vi "CopyVI.vi"(8 "error in (no error)":errorcluster, 9 "application reference (local)":refnum<vi>, 10 "Empty File":path=path "D:/Git/CSPP_MessageMaker/_CSPP_MessageMaker/TestVIs/TestTarget.vi", 11 "File to Copy":path) -> (0 "error out":errorcluster)   [LabVIEW 2014]
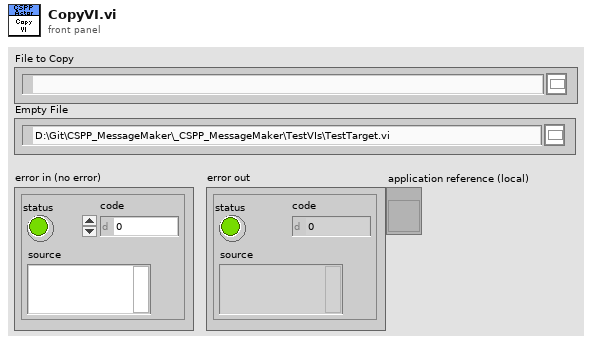
[diagram p1: front panel]
types:
  T1 = enum16{"Invalid Wire Rule", "Required", "Recommended", "Optional", "Dynamic Dispatch"}
  T2 = enum16{"Invalid Wire Rule", "Required", "Recommended", "Optional", "Dynamic Dispatch"}[]
  T3 = typedef "LVPositionTypeDef.ctl" = cluster{"Left":i32, "Top":i32}
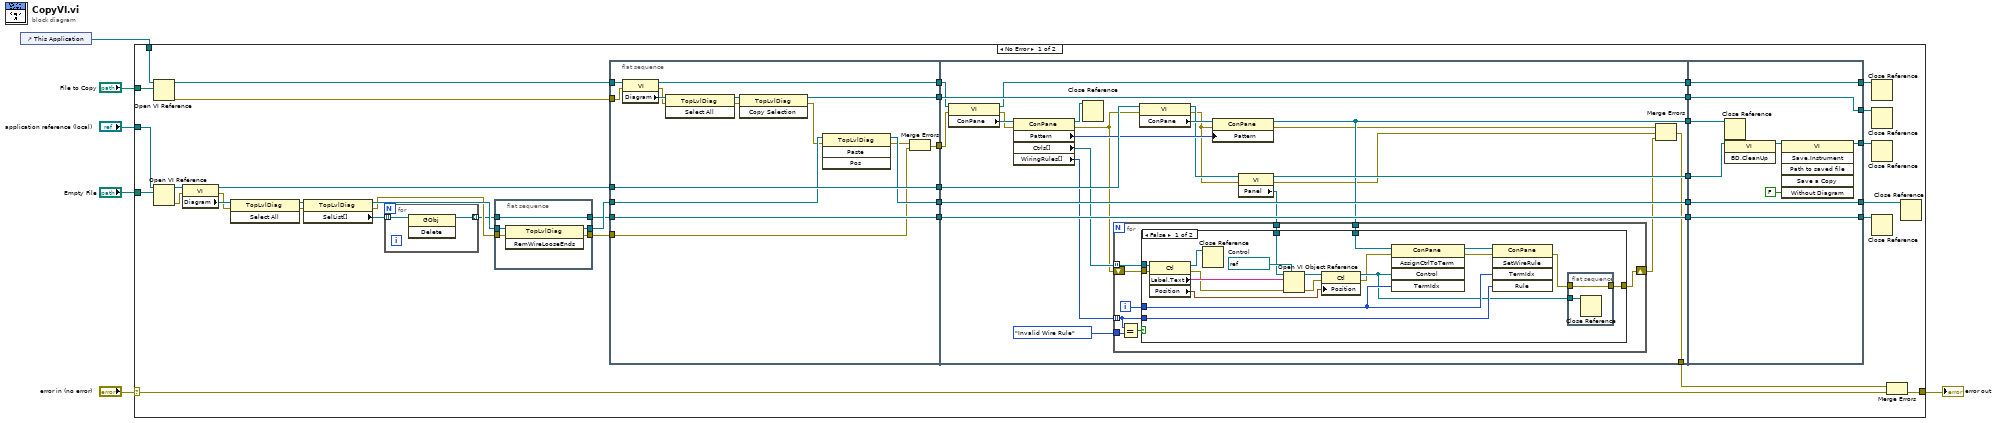
[diagram p0: block diagram]
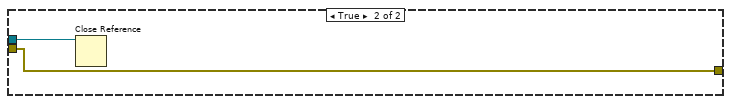
[diagram p2: hidden frame]
diagram:
  n1 = control-ref of="This Application"() -> (w1:refnum<vi>)
  n2 = case shown="No Error" "error in (no error)" {
    selector: "error in (no error)" -> [w13 w136]
    tunnel: [w12 w136] -> w5
    tunnel: "File to Copy" -> [w19 _]
    tunnel: "Empty File" -> [w18 _]
    tunnel: "application reference (local)" -> [w16 _]
    tunnel: w1 -> [w7 _]
    frame No Error {
      n3 = Open VI Reference(application reference (local)=w7, vi path=w19) -> (vi reference=w29:refnum<vi>, error out=w28:errorcluster)  [unwired: 4 in]
      n4 = Open VI Reference(application reference (local)=w16, vi path=w18) -> (vi reference=w35:refnum<vi>, error out=w30:errorcluster)  [unwired: 4 in]
      n5 = property class="VI"(reference=w35, error in=w30) -> (reference out=w27:refnum<vi>, error out=w33:errorcluster, "Diagram"=w34:refnum<vi>)
      n6 = invoke class="TopLvlDiag" method="Select All"(reference=w34, error in=w33) -> (reference out=w32:refnum<vi>, error out=w31:errorcluster)  [unwired: 1 in, 1 out]
      n7 = property class="TopLvlDiag"(reference=w32, error in=w31) -> (reference out=w21:refnum<vi>, error out=w10:errorcluster, "SelList[]"=w17:refnum<vi>[])
      n8 = for {
        tunnel: w17 -> [w135] mode=indexing
        tunnel: [w134] -> w8 mode=indexing
        n9 = invoke class="GObj" method="Delete"(reference=w135) -> (reference out=w134:refnum<vi>)  [unwired: 2 in, 2 out]
      }
      n10 = flat-sequence {
        tunnel: w21 -> [w51]
        tunnel: [w50] -> w20
        tunnel: [w49] -> w15
        tunnel: w10 -> [w48]
        tunnel: [w47] -> w9
        tunnel: w8 -> [w47]
        frame #0 {
          n11 = invoke class="TopLvlDiag" method="RemWireLooseEnds"(reference=w51, error in=w48) -> (reference out=w50:refnum<vi>, error out=w49:errorcluster)  [unwired: 1 in, 1 out]
        }
      }
      n12 = flat-sequence {
        tunnel: w29 -> [w67]
        tunnel: w28 -> [w66]
        tunnel: w20 -> [w59]
        tunnel: w9 -> [w61]
        tunnel: w27 -> [w60]
        tunnel: [w58] -> w46
        tunnel: [w61] -> w45
        tunnel: [w60] -> w44
        tunnel: [w56] -> w43
        tunnel: [w53] -> w42
        tunnel: w15 -> [w54]
        tunnel: [w52] -> w14
        tunnel: w46 -> [w86]
        tunnel: [w86] -> w41
        tunnel: w45 -> [w92]
        tunnel: [w92] -> w40
        tunnel: w44 -> [w85]
        tunnel: [w79] -> w39
        tunnel: w43 -> [w89]
        tunnel: [w88] -> w38
        tunnel: w42 -> [w91]
        tunnel: [w91] -> w37
        tunnel: [w77] -> w36
        tunnel: w14 -> [w76]
        tunnel: [w69] -> w11
        tunnel: [w132] -> w25
        tunnel: [w133] -> w26
        tunnel: w41 -> [w133]
        tunnel: w40 -> [w132]
        tunnel: w39 -> [w130]
        tunnel: [w129] -> w24
        tunnel: [w128] -> w23
        tunnel: w38 -> [w128]
        tunnel: [w127] -> w22
        tunnel: w37 -> [w127]
        tunnel: w36 -> [w126]
        frame #0 {
          n13 = property class="VI"(reference=w67, error in=w66) -> (reference out=w56:refnum<vi>, error out=w64:errorcluster, "Diagram"=w65:refnum<vi>)
          n14 = invoke class="TopLvlDiag" method="Select All"(reference=w65, error in=w64) -> (reference out=w63:refnum<vi>, error out=w62:errorcluster)  [unwired: 1 in, 1 out]
          n15 = invoke class="TopLvlDiag" method="Copy Selection"(reference=w63, error in=w62) -> (reference out=w53:refnum<vi>, error out=w57:errorcluster)  [unwired: 1 in, 1 out]
          n16 = invoke class="TopLvlDiag" method="Paste"(reference=w59, error in=w57) -> (reference out=w58:refnum<vi>, error out=w55:errorcluster)  [unwired: 2 in, 2 out]
          n17 = Merge Errors(w55, w54) -> (w52:errorcluster)
        }
        frame #1 {
          n18 = property class="VI"(reference=w89, error in=w76) -> (reference out=w88:refnum<vi>, error out=w75:errorcluster, "ConPane"=w90:refnum<vi>)
          n19 = property class="ConPane"(reference=w90, error in=w75) -> (reference out=w84:refnum<vi>, error out=w73:errorcluster, "Pattern"=w83:u32, "Ctrls[]"=w82:refnum<vi>[], "WiringRules[]"=w81:T2)
          n20 = Close Reference(reference=w84) -> ()  [unwired: 1 in, 1 out]
          n21 = property class="VI"(reference=w85, error in=w73) -> (reference out=w80:refnum<vi>, error out=w74:errorcluster, "ConPane"=w87:refnum<vi>)
          n22 = property class="ConPane"(reference=w87, error in=w74, "Pattern"=w83) -> (reference out=w77:refnum<vi>, error out=w70:errorcluster)
          n23 = property class="VI"(reference=w80, error in=w74) -> (reference out=w79:refnum<vi>, error out=w71:errorcluster, "Panel"=w78:refnum<vi>)
          n24 = for {
            tunnel: w82 -> [w101] mode=indexing
            tunnel: w81 -> [w95] mode=indexing
            tunnel: w78 -> [w100]
            tunnel: w77 -> [w99]
            shift-right: [w97] -> w72
            shift-left: w73 -> [w98]
            tunnel: T1."Invalid Wire Rule" ("Wire Rule") -> [w93]
            i -> [w96]
            n25 = Equal?(x=w95, y=w93) -> (x = y?=w94:bool)
            n26 = case shown="False" w94 {
              tunnel: w101 -> [w120 w124]
              tunnel: w100 -> [w117 _]
              tunnel: w99 -> [w112 _]
              tunnel: w96 -> [w111 _]
              tunnel: w95 -> [w110 _]
              tunnel: w98 -> [w107 w123]
              tunnel: [w102 w123] -> w97
              frame False {
                w118 = refnum<vi> refnum  # Control
                n27 = property class="Ctl"(reference=w120, error in=w107) -> (reference out=w119:refnum<vi>, error out=w106:errorcluster, "Label.Text"=w116:string, "Position"=w114:T3)
                n28 = Close Reference(reference=w119) -> ()  [unwired: 1 in, 1 out]
                n29 = Open VI Object Reference(7:w118, 8:w106, 10:w116, 11:w117) -> (0:w105:errorcluster, 3:w115:refnum<vi>)
                n30 = property class="Ctl"(reference=w115, error in=w105, "Position"=w114) -> (reference out=w109:refnum<vi>, error out=w104:errorcluster)
                n31 = invoke class="ConPane" method="AssignCtrlToTerm"(reference=w112, error in=w104, "Control"=w109, "TermIdx"=w111) -> (reference out=w113:refnum<vi>, error out=w103:errorcluster)  [unwired: 1 in, 3 out]
                n32 = invoke class="ConPane" method="SetWireRule"(reference=w113, error in=w103, "TermIdx"=w111, "Rule"=w110) -> (error out=w108:errorcluster)  [unwired: 1 in, 4 out]
                n33 = flat-sequence {
                  tunnel: w109 -> [w122]
                  tunnel: w108 -> [w121]
                  tunnel: [w121] -> w102
                  frame #0 {
                    n34 = Close Reference(reference=w122) -> ()  [unwired: 1 in, 1 out]
                  }
                }
              }
              frame True {
                n35 = Close Reference(reference=w124) -> ()  [unwired: 1 in, 1 out]
              }
            }
          }
          n36 = Merge Errors(w70, w71, w72) -> (w69:errorcluster)
        }
        frame #2 {
          n37 = Close Reference(reference=w126) -> ()  [unwired: 1 in, 1 out]
          n38 = invoke class="VI" method="BD.CleanUp"(reference=w130) -> (reference out=w131:refnum<vi>)  [unwired: 2 in, 2 out]
          n39 = invoke class="VI" method="Save.Instrument"(reference=w131, "Without Diagram"=FALSE) -> (reference out=w129:refnum<vi>)  [unwired: 4 in, 5 out]
        }
      }
      n40 = Close Reference(reference=w23) -> ()  [unwired: 1 in, 1 out]
      n41 = Close Reference(reference=w22) -> ()  [unwired: 1 in, 1 out]
      n42 = Close Reference(reference=w24) -> ()  [unwired: 1 in, 1 out]
      n43 = Close Reference(reference=w25) -> ()  [unwired: 1 in, 1 out]
      n44 = Merge Errors(w11, w13) -> (w12:errorcluster)
      n45 = Close Reference(reference=w26) -> ()  [unwired: 1 in, 1 out]
    }
    frame Error {
    }
  }
  "error out" <- w5
